vi "Run.vi"(7 "Team Index":i32, 8 "Column":i32, 9 "Row":i32, 10 "View":i32[](array[numeric]) caption="View (Team Index, -1: empty)", 11 "Coward In":refnum<class "Coward.lvclass">) -> (0 "Replicated":refnum<class "Square.lvclass">, 1 "Direction":T1, 2 "Action":T2, 3 "Coward Out":refnum<class "Coward.lvclass">)   [LabVIEW 2015, in "Coward.lvclass"]
uses:
  Coward.lvclass
  Type Defs/Action Enum.ctl
  Type Defs/Direction Enum.ctl
  Square/Square.lvclass
  Carl/Formics/Attack Options.ctl
  Carl/Common/Reverse Direction.vi
  Carl/Common/Common.lvlib
  Carl/Formics/Formics.lvclass
  Type Defs/SB Type Defs.lvlib
panel:
  # "NW\nN\nNE\nE\nSE\nS\nSW\nW"
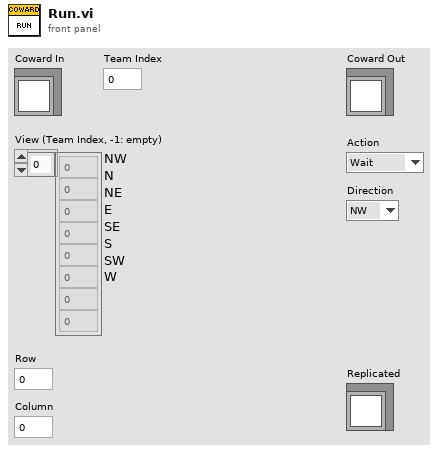
[diagram p1: front panel]
types:
  T1 = typedef "SB Type Defs.lvlib/Direction Enum.ctl" = enum16{"NW", "N", "NE", "E", "SE", "S", "SW", "W"}
  T2 = typedef "SB Type Defs.lvlib/Action Enum.ctl" = enum16{"Wait", "Move", "Attack", "Replicate"}
  T3 = typedef "Formics.lvclass/Attack Options.ctl" = enum16{"Attack", "Run", "Distract"}
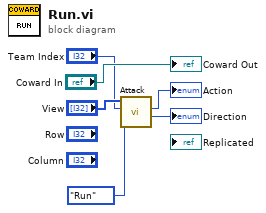
[diagram p0: block diagram]
diagram:
  n1 = call "Attack.vi"("Attack?"=Attack_Options."Run", "Team Index"="Team Index", "View"="View") -> ("Direction"=→"Direction":i32, "Action"=→"Action":T2)  [unwired: 3 in, 4 out]
  "Coward Out" <- "Coward In"
